vi "CS_cRIO-PB_MSAC2_DPV1-WriteReq.vi"(0 "FPGA VI Reference":T7, 5 "Slave":i8, 7 "Write data":T5 {"Slot number:" format="%0.0f"; "Communication ref.:" format="%0.0f"; "Data:" format="%.0x"}, 11 "Error":errorcluster) -> (4 "FPGA VI Reference out":T7, 6 "Result":T6, 8 "Write response data":T1 {"Error data"."Error decode:" format="%.0x"; "Error data"."Remote address:" format="%0.0f"; "Error data"."Communication ref.:" format="%0.0f"; "Abort data"."Reasoncode:" format="%.0x"; "Abort data"."Instance:" format="%.0x"; "Abort data"."Additional detail:" format="%04x"; "Abort data"."Subnet:" format="%.0x"; "Abort data"."Response SAP:" format="%0.0f"; "Abort data"."Remote address:" format="%0.0f"; "Write data"."Communication ref.:" format="%0.0f"}, 15 "Error out":errorcluster)   [LabVIEW 2013, in "dynamic profibus.lvlib"]
doc: "Handles the cyclic process data of the selected DP-Slave.\n\nFPGA VI Reference:\nReference of the FPGA VI.\n\nSlave:\nPROFIBUS address of the DP-Slave. \n\nModify output data:\nThe Modify output data array contains the DP-Slave output data to be changed.\n\nInput data:\nThe Input data array contains the DP-Slave input data.\n\nOutput data:\nThe Output data array contains the DP-Slave output data.\n\nInput length:\nReturns the configured input length of the DP-Slave.\n\nOutput length:\nReturns the configured output length of the DP-Slave.\n\nSlave status:\n0x00: DP-Slave is in DataExchange mode, input and output data are valid\n0xC3: DP-Slave is not in Data Exchange mode, input and output data are invalid, DP-Slave diagnostic data are reported in Diag data array\n0xFF: DP-Slave is in Data Exchange mode and reports ext. diagnostic data, input and output data are valid.\n\nFPGA VI Reference out:\nIs a copy of the FPGA VI Reference .\n\nError in:\nPreceding error conditions. If an error has already occurred, the VI returns the value of the error in Error out.\n\nError out:\nError: TRUE if an error occurred.\nStatus: Error code\nInfo: Error description"
uses:
  dynamic profibus.lvlib
  fpga reference.ctl
  <vilib>/addons/Comsoft.lib/cRIO PBMS/Examples/SubVIs/CS_PB_DPV1_AbortIndData.ctl
  <vilib>/addons/Comsoft.lib/cRIO PBMS/Examples/SubVIs/CS_PB_DPV1_ErrorData.ctl
  <vilib>/addons/Comsoft.lib/cRIO PBMS/Examples/SubVIs/CS_PB_DPV1_Result.ctl
  <vilib>/addons/Comsoft.lib/cRIO PBMS/Examples/SubVIs/CS_PB_DPV1_WriteReqData.ctl
  <vilib>/addons/Comsoft.lib/cRIO PBMS/Examples/SubVIs/CS_PB_DPV1_WriteConData.ctl
  <vilib>/addons/Comsoft.lib/cRIO PBMS/Examples/SubVIs/CS_PB_DPV1_WriteResData.ctl
panel:
  # "The DPV1 variables of a DP Slave are selected by the parameters Slot number and Index. Refer to the documentation of the DP Slave for a detailed description of all available variables."
  # "-Enter the identical value (1) for Communication ref as used for InitateReq.\n\n- Enter the Slot Number, Index, Data and Length for the DPV1 variable to be written. To enter the DP Slave address is not necessary; this is decoded via the Communication ref parameter, which was assigned as 1 during connection setup.\n\n- Click the DPV1 Write button. After the service is completed, the Result has to display Success, what means that DPV1 data has been successfully written on the DP Slave.\n\nIf the Result does not display Success, check the Abort and Error section. See Context Help for detailed description of error checking."
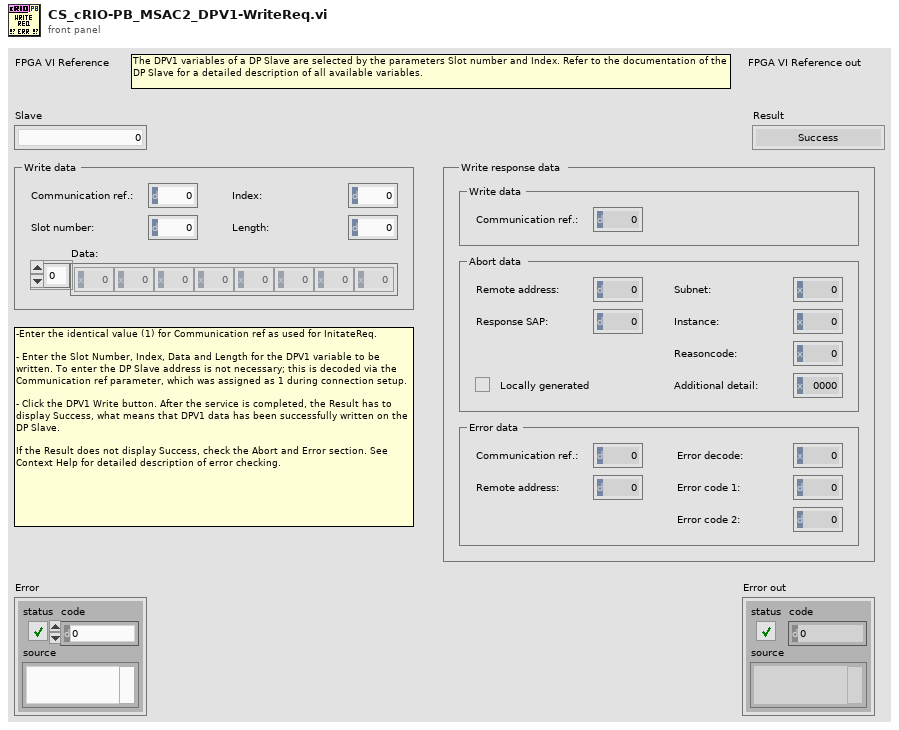
[diagram p1: front panel]
types:
  T1 = typedef "CS_PB_DPV1_WriteResData.ctl" = cluster{"Write data":T2, "Abort data":T3, "Error data":T4}
  T2 = typedef "CS_PB_DPV1_WriteConData.ctl" = cluster{"Communication ref.:":u8}
  T3 = typedef "CS_PB_DPV1_AbortIndData.ctl" = cluster{"Remote address:":u8, "Response SAP:":u8, "Locally generated":bool, "Subnet:":u8, "Instance:":u8, "Reasoncode:":u8, "Additional detail:":u16}
  T4 = typedef "CS_PB_DPV1_ErrorData.ctl" = cluster{"Communication ref.:":u8, "Remote address:":u8, "Error decode:":u8, "Error code 1:":u8, "Error code 2:":u8}
  T5 = typedef "CS_PB_DPV1_WriteReqData.ctl" = cluster{"Communication ref.:":u8, "Slot number:":u8, "Index:":u8, "Length:":u8, "Data:":u8[]}
  T6 = typedef "CS_PB_DPV1_Result.ctl" = enum16{"Success", "Abort", "Error"}
  T7 = typedef "dynamic profibus.lvlib/fpga reference.ctl" = refnum<k20>
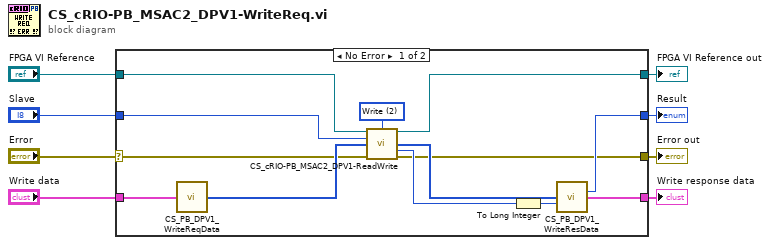
[diagram p0: block diagram]
diagram:
  n1 = case shown="No Error" "Error" {
    selector: "Error" -> [w16 w22]
    tunnel: "Slave" -> [w12 _]
    tunnel: "FPGA VI Reference" -> [w14 w23]
    tunnel: [w15 w23] -> w1
    tunnel: [w17 w22] -> w3
    tunnel: [w10 _] -> w4
    tunnel: [w19 _] -> w2
    tunnel: "Write data" -> [w9 _]
    frame No Error {
      w13 = i8 2 items=["Initiate", "Read", "Write", "Abort"] ("DPV1-Service")
      n2 = call <vilib>:"CS_PB_DPV1_WriteReqData.vi"("Write data"=w9) -> ("Request data"=w20:u8[])  [unwired: 14 in]
      n3 = call "CS_cRIO-PB_MSAC2_DPV1-ReadWrite.vi"("FPGA VI Reference"=w14, "DPV1-Service"=w13, "Slave"=w12, "Data"=w20, "Error"=w16) -> ("FPGA VI Reference out"=w15:T7, "Data out"=w21:u8[], "Status"=w18:u8, "Error out"=w17:errorcluster)  [unwired: 7 in]
      n4 = To Long Integer(number=w18) -> (32bit integer=w11:i32)
      n5 = call <vilib>:"CS_PB_DPV1_WriteResData.vi"("Response data"=w21, "Status"=w11) -> ("Result"=w19:T6, "Write response data"=w10:T1)  [unwired: 12 in]
    }
    frame Error {
    }
  }
  "Error out" <- w3
  "FPGA VI Reference out" <- w1
  "Result" <- w2
  "Write response data" <- w4
